vi "Read Steps From File.vi"(11 "configuration file path":path) -> (0 "error out":errorcluster, 3 "Step Data Array":T1[](array[typedef]))   [LabVIEW 2011]
uses:
  HelperVIs.llb/StepData.ctl
  HelperVIs.llb/StepProperties.ctl
  <vilib>/Utility/config.llb/Read Key (String).vi
  <vilib>/Utility/config.llb/NI_LVConfig.lvlib
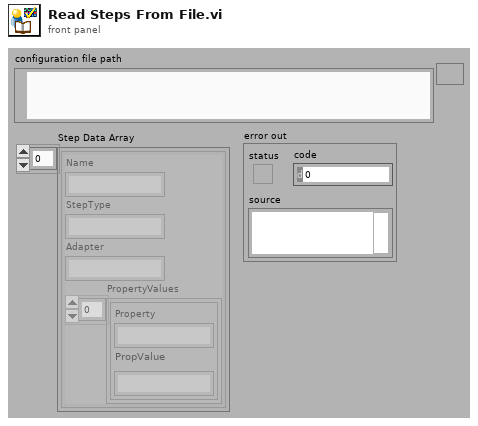
[diagram p1: front panel]
types:
  T1 = typedef "StepData.ctl" = cluster{"Name":string, "StepType":string, "Adapter":string, "PropertyValues":T2[]}
  T2 = typedef "StepProperties.ctl" = cluster{"Property":string, "PropValue":string}
  T3 = typedef "NI_LVConfig.lvlib/Config Data RefNum.ctl" = refnum<k1>
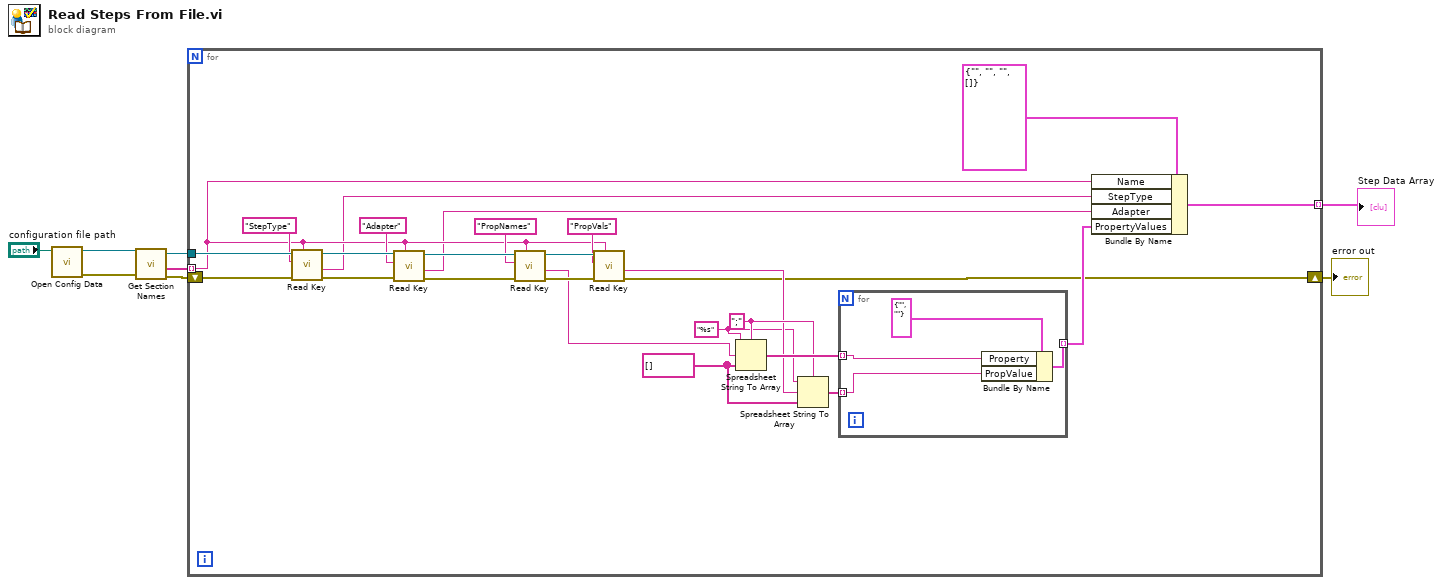
[diagram p0: block diagram]
diagram:
  n1 = call <vilib>:"Open Config Data.vi"("configuration file path"="configuration file path") -> ("error out"=w5:errorcluster, "refnum"=w8:T3)  [unwired: 8 in, 1 out]
  n2 = call <vilib>:"Get Section Names.vi"("error in (no error)"=w5, "refnum"=w8) -> ("error out"=w2:errorcluster, "section names"=w6:string[], "refnum out"=w7:T3)  [unwired: 7 in]
  n3 = for {
    tunnel: w7 -> [w34]
    tunnel: w6 -> [w19] mode=indexing
    tunnel: [w15] -> w4 mode=indexing
    shift-right: [w10] -> w1
    shift-left: w2 -> [w9]
    w12 = "%s" ("format string")
    w21 = ";" ("delimiter (Tab)")
    w11 = string[] []
    n4 = call-poly <vilib>:"Read Key.vi"("section"=w19, "error in (no error)"=w9, "key"="StepType", "refnum"=w34) -> ("error out"=w28:errorcluster, "value"=w18:string, "refnum out"=w32:T3)  [unwired: 4 in, 1 out]
    n5 = call-poly <vilib>:"Read Key.vi"("section"=w19, "error in (no error)"=w28, "key"="Adapter", "refnum"=w32) -> ("error out"=w27:errorcluster, "value"=w17:string, "refnum out"=w31:T3)  [unwired: 4 in, 1 out]
    n6 = call-poly <vilib>:"Read Key.vi"("section"=w19, "error in (no error)"=w27, "key"="PropNames", "refnum"=w31) -> ("error out"=w24:errorcluster, "value"=w14:string, "refnum out"=w26:T3)  [unwired: 4 in, 1 out]
    n7 = call-poly <vilib>:"Read Key.vi"("section"=w19, "error in (no error)"=w24, "key"="PropVals", "refnum"=w26) -> ("error out"=w10:errorcluster, "value"=w13:string)  [unwired: 4 in, 2 out]
    n8 = Spreadsheet String To Array(delimiter (Tab)=w21, format string=w12, spreadsheet string=w14, array type (2D Dbl)=w11) -> (array=w22:string[])
    n9 = Spreadsheet String To Array(delimiter (Tab)=w21, format string=w12, spreadsheet string=w13, array type (2D Dbl)=w11) -> (array=w23:string[])
    n10 = for {
      tunnel: w23 -> [w36] mode=indexing
      tunnel: w22 -> [w37] mode=indexing
      tunnel: [w35] -> w16 mode=indexing
      n11 = Bundle By Name(cluster=T2 {"Property"="", "PropValue"=""} ("Property Data"), "Property"=w37, "PropValue"=w36) -> (w35:T2)
    }
    n12 = Bundle By Name(cluster=T1 {"Name"="", "StepType"="", "Adapter"="", "PropertyValues"=[]} ("Step Data"), "Name"=w19, "StepType"=w18, "Adapter"=w17, "PropertyValues"=w16) -> (w15:T1)
  }
  "Step Data Array" <- w4
  "error out" <- w1
